vi "CheckIfPlaceholder.vi"(8 "error in (no error)":errorcluster, 11 "Data":variant) -> (0 "error out":errorcluster, 2 "IsPlacerholder?":bool, 3 "Data (dup)":variant)   [LabVIEW 2019, in "BlueSerialization.lvlib" / "BlueSerializer.lvclass"]
uses:
  BlueSerializer.lvclass
  <vilib>/Utility/Data Type/Type Definitions/Data Type.ctl
  <vilib>/Utility/Data Type/NI_Data Type.lvlib
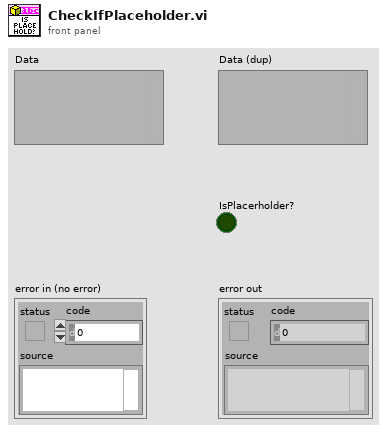
[diagram p1: front panel]
types:
  T1 = typedef "NI_Data Type.lvlib/Data Type.ctl" = enum8{"Invalid Type", "Void", "I8", "I16", "I32", "I64", "U8", "U16", "U32", "U64", "Single Float", "Double Float", "Extended Float", "Single Complex", "Double Complex", "Extended Complex", "Enum U8", "Enum U16", "Enum U32", "Enum U64", "Single Float With Unit", "Double Float With Unit", "Extended Float With Unit", "Single Complex with Unit", "Double Complex with Unit", "Extended Complex with Unit", "Boolean", "String", "Path", "Picture", "Tag", "Array", "Cluster", "Variant", "LV Variant", "Waveform", "Timestamp", "Digital Waveform", "Digital Data", "ExpressData", "Refnum", "External Data", "VI", "Poly VI", "LabVIEW Class Instance", "Fixed Point", "Set Collection", "Map Collection"}
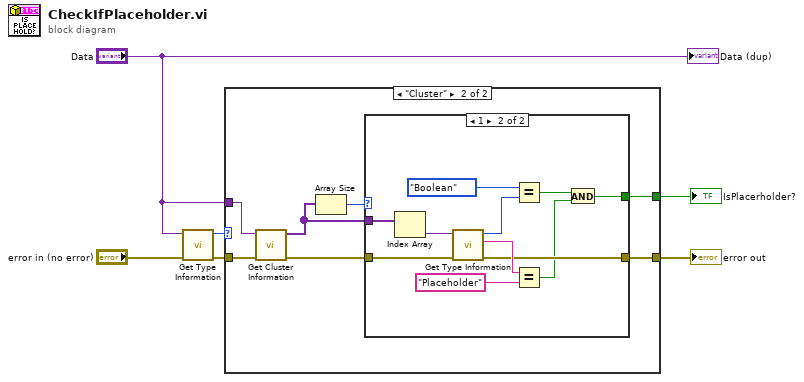
[diagram p0: block diagram]
diagram:
  n1 = call <vilib>:"Get Type Information.vi"("error in (no error)"="error in (no error)", "variant"="Data") -> ("error out"=w3:errorcluster, "type"=w2:T1)  [unwired: 5 in, 3 out]
  n2 = case shown="\"Cluster\"" w2 {
    tunnel: "Data" -> [_ w14]
    tunnel: [_ w11] -> w6
    tunnel: w3 -> [w7 w10]
    tunnel: [w7 w8] -> w5
    frame Default {
      # "Not a cluster so return false."
    }
    frame "Cluster" {
      n3 = call <vilib>:"Get Cluster Information.vi"("error in (no error)"=w10, "variant"=w14) -> ("error out"=w9:errorcluster, "cluster elements"=w12:variant[])  [unwired: 8 in]
      n4 = Array Size(array=w12) -> (size(s)=w13:i32)
      n5 = case shown="1" w13 {
        tunnel: w12 -> [_ w26]
        tunnel: [_ w16] -> w11
        tunnel: w9 -> [w15 w25]
        tunnel: [w15 w19] -> w8
        frame Default {
          # "Cluster does not have the right number of elements."
        }
        frame 1 {
          n6 = Index Array(array=w26) -> (element=w24:variant)  [unwired: 1 in]
          n7 = call <vilib>:"Get Type Information.vi"("error in (no error)"=w25, "variant"=w24) -> ("error out"=w19:errorcluster, "name"=w21:string, "type"=w23:T1)  [unwired: 5 in, 2 out]
          n8 = Equal?(x=Data_Type."Boolean" ("Type"), y=w23) -> (x = y?=w18:bool)
          n9 = Equal?(x=w21, y="Placeholder") -> (x = y?=w17:bool)
          n10 = And(x=w18, y=w17) -> (x .and. y?=w16:bool)
        }
      }
    }
  }
  "IsPlacerholder?" <- w6
  "error out" <- w5
  "Data (dup)" <- "Data"
